vi "sum_for_multiple.vi"(2 "B":T1, 3 "A":T3) -> (0 "Output":T2, 1 "Y0":bool)   [LabVIEW 2013]
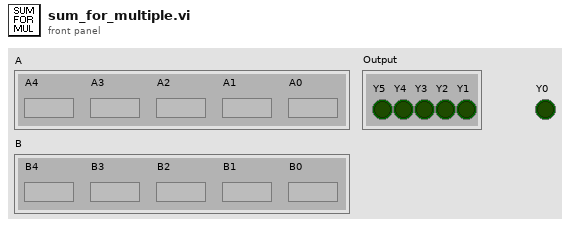
[diagram p1: front panel]
types:
  T1 = cluster{"B4":bool, "B3":bool, "B2":bool, "B1":bool, "B0":bool}
  T2 = cluster{"Y4":bool, "Y3":bool, "Y2":bool, "Y1":bool, "Y5":bool}
  T3 = cluster{"A4":bool, "A3":bool, "A2":bool, "A1":bool, "A0":bool}
  T4 = cluster{"C":bool, "S":bool, "S":bool, "S":bool, "S":bool}
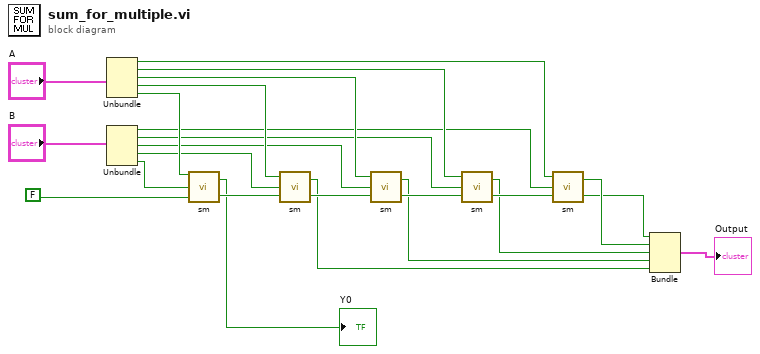
[diagram p0: block diagram]
diagram:
  n1 = Unbundle("A") -> ("A4"=w13:bool, "A3"=w14:bool, "A2"=w15:bool, "A1"=w16:bool, "A0"=w18:bool)
  n2 = Unbundle("B") -> ("B4"=w9:bool, "B3"=w10:bool, "B2"=w11:bool, "B1"=w12:bool, "B0"=w17:bool)
  n3 = call "sm.vi"("c"=FALSE, "b"=w17, "a"=w18) -> ("C"=w19:bool, "S"=→"Y0":bool)
  n4 = call "sm.vi"("c"=w19, "b"=w12, "a"=w16) -> ("C"=w20:bool, "S"=w8:bool)
  n5 = call "sm.vi"("c"=w20, "b"=w11, "a"=w15) -> ("C"=w21:bool, "S"=w7:bool)
  n6 = call "sm.vi"("c"=w21, "b"=w10, "a"=w14) -> ("C"=w22:bool, "S"=w6:bool)
  n7 = call "sm.vi"("c"=w22, "b"=w9, "a"=w13) -> ("C"=w1:bool, "S"=w5:bool)
  n8 = Bundle("C"=w1, "S"=w5, "S"=w6, "S"=w7, "S"=w8) -> (→"Output":T4)  [unwired: 1 in]
